vi "System Exec(old).vi"(5 "expected output size  (4096)":u32=4096, 6 "run minimized? (F)":bool, 7 "wait until completion? (T)":bool=TRUE, 8 "error in (no error)":errorcluster, 9 "working directory":path=path "", 10 "standard input":string, 11 "command line":string) -> (0 "error out":errorcluster, 1 "return code":i32, 2 "standard error":string, 3 "standard output":string)   [LabVIEW 2021]
doc: "Executes a system command."
panel:
  in  "error string (in control for localization)":string="System Exec.vi. Command was \"%s\""
  # "Note:  If wait until completion?\nis False, standard input, output,\nand error will be ignored."
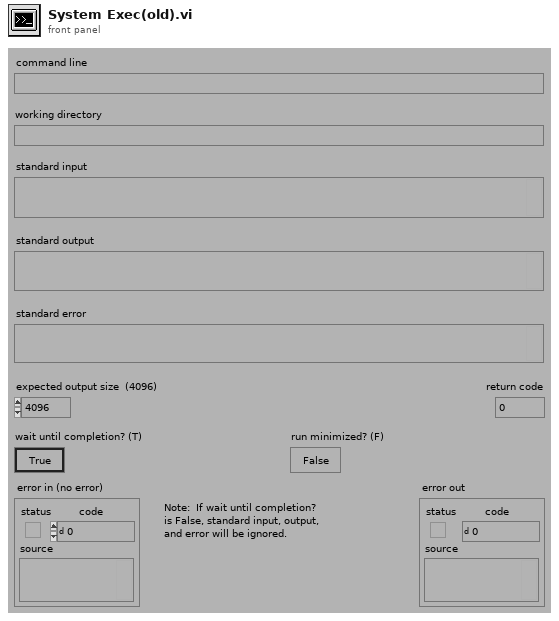
[diagram p1: front panel]
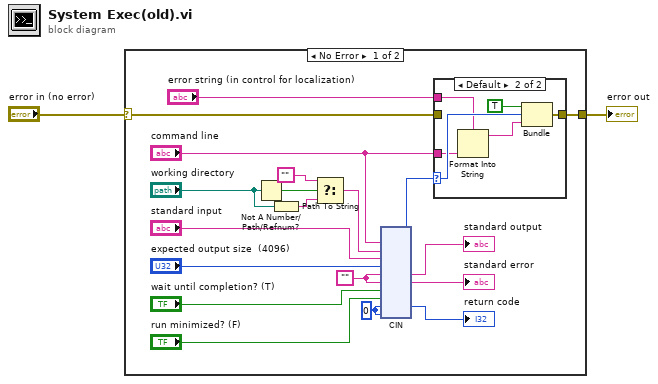
[diagram p0: block diagram]
diagram:
  n1 = case shown="No Error" "error in (no error)" {
    selector: "error in (no error)" -> [w14 w29]
    tunnel: [w13 w29] -> w1
    frame No Error {
      w8 = 0 ("Input Value")
      w19 = ""
      n2 = Not A Number/Path/Refnum?(number/path/refnum="working directory") -> (NaN/Path/Refnum?=w6:bool)
      n3 = Path To String(path="working directory") -> (string=w3:string)
      n4 = Select(t="", s=w6, f=w3) -> (s? t:f=w5:string)
      n5 = cin("command line", w5, "standard input", "expected output size  (4096)", w19, w19, "wait until completion? (T)", "run minimized? (F)", w8, w8) -> (→"standard output":string, →"standard error":string, →"return code":i32, w9:i32)  [unwired: 6 in]
      n6 = case shown="Default" w9 {
        selector: w9 -> [_ w28]
        tunnel: w14 -> [w22 _]
        tunnel: [w22 w26] -> w13
        tunnel: "command line" -> [_ w25]
        tunnel: "error string (in control for localization)" -> [_ w23]
        frame 0 {
        }
        frame Default {
          n7 = Format Into String(format string=w23, w25) -> (resulting string=w24:string)  [unwired: 2 in, 1 out]
          n8 = Bundle(TRUE, "Input Value"=w28, w24) -> (w26:cluster{bool, "Input Value":i32, string})  [unwired: 1 in]
        }
      }
    }
    frame Error {
    }
  }
  "error out" <- w1
